vi "Cleanup Session.vi"(8 "error in":errorcluster, 11 "Plugin in":refnum<class "Historical Table.lvclass">) -> (0 "error out":errorcluster, 3 "Plugin out":refnum<class "Historical Table.lvclass">)   [LabVIEW 2024, in "Historical Table.lvlib" / "Historical Table.lvclass"]
uses:
  Historical Table.lvclass
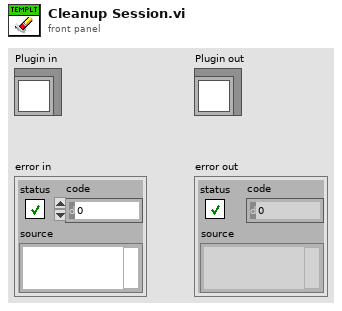
[diagram p1: front panel]
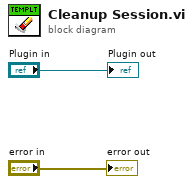
[diagram p0: block diagram]
diagram:
  "error out" <- "error in"
  "Plugin out" <- "Plugin in"
